vi "Generate B-Scan Coordinates.vi"(8 "Error In":errorcluster, 11 "Thorlabs OCT Scan Parameters [in]":T1={"Index of Refraction"=1.0, "Columns"=1000, "Range X [mm]"=2.0, "B-Scan Averaging"=1, "BScan X offset [mm]"=0.0, "BScan Y offset [mm]"=0.0, "BScan angle [deg]"=0.0, "Window"=enum."Hann", "Spectral Ave."=0, "A-Scan Ave."=0} {"BScan Y offset [mm]" min=-5.0 max=5.0 format="%_4f"; "BScan X offset [mm]" min=-5.0 max=5.0 format="%_4f"; "B-Scan Averaging" min=1 max=20 step=1; "Range X [mm]" min=0.0 max=10.0 step=0.5 format="%_3f"; "Columns" min=50 max=10240 step=1; "Index of Refraction" min=1.0 max=5.0 step=0.10000000149011612 format="%.3f"}) -> (0 "Error Out":errorcluster, 1 "End Coordinates":cluster{"Start X":dbl, "Start Y":dbl}, 2 "Start Coordinates":cluster{"Start X":dbl, "Start Y":dbl}, 3 "Thorlabs OCT Scan Parameters [out]":T1={"Index of Refraction"=1.0, "Columns"=1000, "Range X [mm]"=2.0, "B-Scan Averaging"=1, "BScan X offset [mm]"=0.0, "BScan Y offset [mm]"=0.0, "BScan angle [deg]"=0.0, "Window"=enum."Hann", "Spectral Ave."=0, "A-Scan Ave."=0} {"BScan Y offset [mm]" min=-5.0 max=5.0 format="%_4f"; "BScan X offset [mm]" min=-5.0 max=5.0 format="%_4f"; "B-Scan Averaging" min=1 max=20 step=1; "Range X [mm]" min=0.0 max=10.0 step=0.5 format="%_3f"; "Columns" min=50 max=10240 step=1; "Index of Refraction" min=1.0 max=5.0 step=0.10000000149011612 format="%.3f"}, 5 "Num A-Lines":i32)   [LabVIEW 2017]
uses:
  Controls/ThorlabsOCT Scan Parameters.ctl
  user.lib/SpectralRadar.llb/Scan Pattern.lvclass
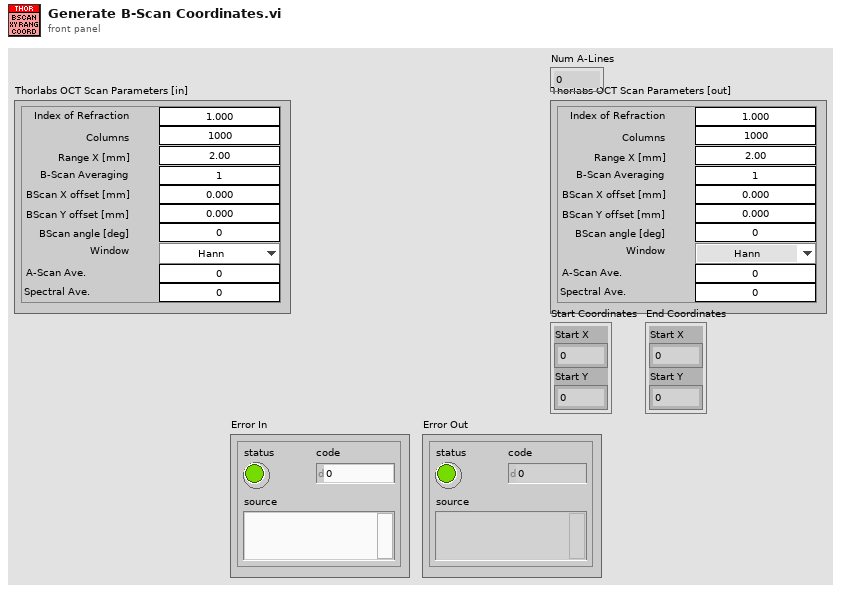
[diagram p1: front panel]
types:
  T1 = typedef "ThorlabsOCT Scan Parameters.ctl" = cluster{"Index of Refraction":dbl, "Columns":i32, "Range X [mm]":dbl, "B-Scan Averaging":i32, "BScan X offset [mm]":dbl, "BScan Y offset [mm]":dbl, "BScan angle [deg]":dbl, "Window":enum16{"Hann", "Hamming", "Gauss", "Tapered Cosine", "Blackman", "4 Term B-Harris"}, "Spectral Ave.":i32, "A-Scan Ave.":i32}
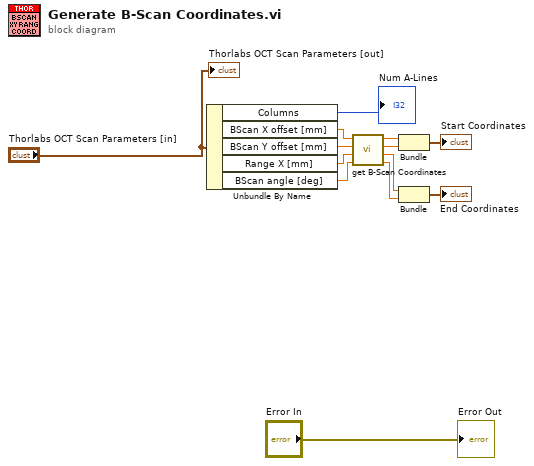
[diagram p0: block diagram]
diagram:
  n1 = Unbundle By Name("Thorlabs OCT Scan Parameters [in]") -> ("Columns"=→"Num A-Lines":i32, "BScan X offset [mm]"=w12:dbl, "BScan Y offset [mm]"=w11:dbl, "Range X [mm]"=w10:dbl, "BScan angle [deg]"=w9:dbl)
  n2 = call "get B-Scan Coordinates.vi"("BScan Angle"=w9, "BScan Range"=w10, "Offset Y"=w11, "Offset X"=w12) -> ("End Y"=w5:dbl, "End X"=w6:dbl, "Start Y"=w7:dbl, "Start X"=w8:dbl)
  n3 = Bundle("Start X"=w8, "Start Y"=w7) -> (→"Start Coordinates":cluster{"Start X":dbl, "Start Y":dbl})  [unwired: 1 in]
  n4 = Bundle("End X"=w6, "End Y"=w5) -> (→"End Coordinates":cluster{"End X":dbl, "End Y":dbl})  [unwired: 1 in]
  "Thorlabs OCT Scan Parameters [out]" <- "Thorlabs OCT Scan Parameters [in]"
  "Error Out" <- "Error In"
